vi "Test Invalid Multiple Channels Registration - Data Type.vi"() -> ()   [LabVIEW 2024]
uses:
  Sift API/Sift Client.lvclass
  Generate Sift Protos/SiftProxy_client/RPC Messages/sift_proxy_v1_ChannelDataType.ctl
  Generate Sift Protos/SiftProxy_client/SiftProxy_client.lvlib
panel:
  out "Success":bool
  out "Error":errorcluster
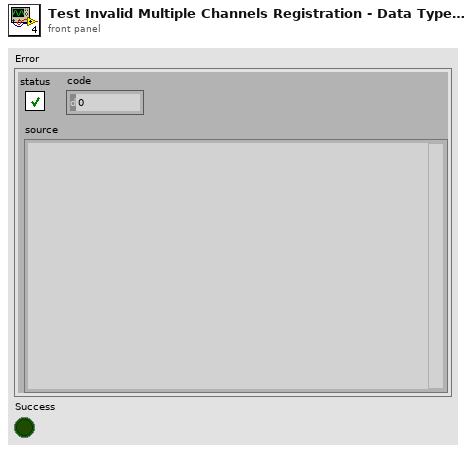
[diagram p1: front panel]
types:
  T1 = typedef "SiftProxy_client.lvlib/sift_proxy_v1_ChannelDataType.ctl" = enum32{"CHANNEL_DATA_TYPE_UNSPECIFIED", "CHANNEL_DATA_TYPE_DOUBLE", "CHANNEL_DATA_TYPE_STRING", "CHANNEL_DATA_TYPE_ENUM", "CHANNEL_DATA_TYPE_BIT_FIELD", "CHANNEL_DATA_TYPE_BOOL", "CHANNEL_DATA_TYPE_FLOAT", "CHANNEL_DATA_TYPE_INT_32", "CHANNEL_DATA_TYPE_UINT_32", "CHANNEL_DATA_TYPE_INT_64", "CHANNEL_DATA_TYPE_UINT_64"}
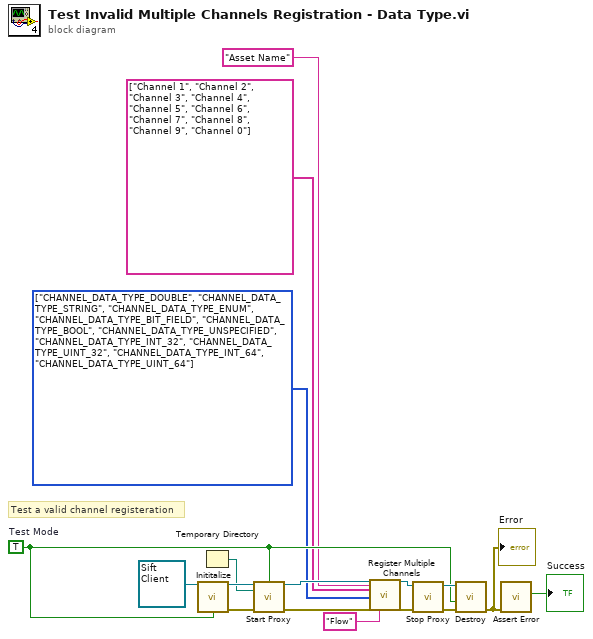
[diagram p0: block diagram]
diagram:
  w4 = T1[] [enum."CHANNEL_DATA_TYPE_DOUBLE", enum."CHANNEL_DATA_TYPE_STRING", enum."CHANNEL_DATA_TYPE_ENUM", enum."CHANNEL_DATA_TYPE_BIT_FIELD", enum."CHANNEL_DATA_TYPE_BOOL", enum."CHANNEL_DATA_TYPE_UNSPECIFIED", enum."CHANNEL_DATA_TYPE_INT_32", enum."CHANNEL_DATA_TYPE_UINT_32", enum."CHANNEL_DATA_TYPE_INT_64", enum."CHANNEL_DATA_TYPE_UINT_64"] items=["CHANNEL_DATA_TYPE_UNSPECIFIED", "CHANNEL_DATA_TYPE_DOUBLE", "CHANNEL_DATA_TYPE_STRING", "CHANNEL_DATA_TYPE_ENUM", "CHANNEL_DATA_TYPE_BIT_FIELD", "CHANNEL_DATA_TYPE_BOOL", "CHANNEL_DATA_TYPE_FLOAT", "CHANNEL_DATA_TYPE_INT_32", "CHANNEL_DATA_TYPE_UINT_32", "CHANNEL_DATA_TYPE_INT_64", "CHANNEL_DATA_TYPE_UINT_64"]
  w11 = TRUE  # Test Mode
  # "Test a valid channel registeration"
  n1 = call-dynamic "Inititalize.vi"("Sift Client in"=refnum<class "Sift Client.lvclass"> refnum ("Sift Client.lvlib:Sift Client.lvclass"), "Test Mode"=w11) -> ("Sift Client out"=w16:refnum<class "Sift Client.lvclass">, "error out"=w15:errorcluster)  [unwired: 12 in]
  n2 = Temporary Directory() -> (w12:path)
  n3 = call-dynamic "Start Proxy.vi"("Sift Client in"=w16, "Test Mode"=w11, "Storage Path"=w12, "error in (no error)"=w15) -> ("Sift Client out"=w10:refnum<class "Sift Client.lvclass">, "error out"=w9:errorcluster)  [unwired: 10 in]
  n4 = call "Register Multiple Channels.vi"("Sift Client in"=w10, "Asset Name"="Asset Name", "Names"=string[] ["Channel 1", "Channel 2", "Channel 3", "Channel 4", "Channel 5", "Channel 6", "Channel 7", "Channel 8", "Channel 9", "Channel 0"], "Data Types"=w4, "error in (no error)"=w9, "Flow Name"="Flow") -> ("Sift Client out"=w7:refnum<class "Sift Client.lvclass">, "error out"=w6:errorcluster)  [unwired: 20 in]
  n5 = call-dynamic "Stop Proxy.vi"("error in (no error)"=w6, "Sift Client in"=w7) -> ("error out"=w14:errorcluster, "Sift Client out"=w13:refnum<class "Sift Client.lvclass">)  [unwired: 7 in, 1 out]
  n6 = call-dynamic "Destroy.vi"("error in (no error)"=w14, "Test Mode"=w11, "Sift Client in"=w13) -> ("error out"=w2:errorcluster)  [unwired: 7 in, 1 out]
  "Error" <- w2
  n7 = call "Assert Error.vi"("Error"=w2) -> ("Success"=→"Success":bool)  [unwired: 10 in]
